vi "Vision_Processing_L_R5.vi"(0 "Current State":T6(ring)=enum."Short Range", 1 "Image Dst":T5=refnum, 2 "Inpute Image":T5=refnum, 3 "Startup Flag":bool, 5 "Current ROI Descriptor":T11={"Global Rectangle"=[0, 0, 320, 240], "Contours"=[{"ID"=enum."External", "Type"=12, "Coordinates"=[0, 0, 320, 240, 0]}]} {"Contours"."Type" items=["No Selection", "Point", "Line", "Rectangle", "Oval", "Polygon", "Freehand Region", "Annulus", "Unused2", "Unused3", "Broken Line", "Freehand Line", "Rotated Rectangle"]}, 6 "Avg Score - Last":dbl=802.5034383138021, 7 "error in (no error)":errorcluster, 8 "Current Settings":T9={"Curve Parameters"={"Extraction Mode"=1, "Edge Threshold"=150, "Edge Filter Size"=0, "Min Length"=25, "Row Search Step Size"=15, "Col Search Step Size"=15, "Max Endpoint Gap"=2, "Closed"=TRUE, "Subpixel"=TRUE}, "Match Mode"={"Rotation"=TRUE, "Scale"=TRUE, "Occlusion"=TRUE, "Reserved"=FALSE, "Reserved"=FALSE, "Reserved"=FALSE}, "Range Settings"=[{"Match Constraints"=0, "Min"=-5.0, "Max"=5.0}, {"Match Constraints"=1, "Min"=20.0, "Max"=150.0}, {"Match Constraints"=2, "Min"=0.0, "Max"=25.0}], "Number of Matches"=1, "Minimum Match Score"=800.0, "SubPixel Accuracy"=TRUE, "Adv. Geometric Match Options 2"=[{"Setup Data Item"=20, "Item Value"=0.0}, {"Setup Data Item"=22, "Item Value"=1.0}]} {"Curve Parameters"."Extraction Mode" items=["Normal", "Uniform Regions"]; "Curve Parameters"."Edge Filter Size" items=["Fine", "Normal", "Contour Tracing"]; "Curve Parameters"."Max Endpoint Gap" min=0; "Curve Parameters"."Col Search Step Size" min=1 max=255 step=1; "Curve Parameters"."Row Search Step Size" min=1 max=255 step=1; "Curve Parameters"."Min Length" min=0; "Curve Parameters"."Edge Threshold" min=1 max=350 step=1; "Range Settings"."Max" format="%.2f"; "Range Settings"."Min" format="%.2f"; "Range Settings"."Match Constraints" items=["Rotation Angle (degrees)", "Scale Factor (%)", "Occlusion (%)"]; "Adv. Geometric Match Options 2"."Setup Data Item" items=["Curve Extraction Mode", "Curve Edge Threshold", "Curve Edge Filter Size", "Min Curve Length", "Curve Row Search Step Size", "Curve Col Search Step Size", "Curve Max Endpoint Gap", "Extract Closed Curves", "Enable Subpixel Curve Extraction", "Enable Correlation Score", "Enable Subpixel Accuracy", "Subpixel Iterations", "Subpixel Tolerance", "Initial Match List Length", "Enable Target Template Curve Score", "Min Match Separation Distance", "Min Match Separation Angle", "Min Match Separation Scale", "Max Match Overlap", "Enable Coarse Result", "Enable Calibration Support", "Enable Contrast Reversal", "Search Strategy", "Refinement Match Factor", "Subpixel Match Factor"]}, 9 "Sub Beacon Search Enable":bool[](array[boolean])=[FALSE, FALSE, FALSE, FALSE, FALSE], 10 "History Data - IN":T4={"Valid Beacon History - in"=[FALSE, FALSE, FALSE, FALSE, FALSE, FALSE, FALSE, FALSE, FALSE, FALSE, FALSE, FALSE, FALSE, FALSE, FALSE, FALSE, FALSE, FALSE, FALSE, FALSE], "Valid Score History"=[916.1194458007812, 0.0, 921.171142578125, 952.2998657226562, 947.6416015625, 946.7607421875, 946.6710815429688, 913.2891235351562, 946.3783569335938, 946.1008911132812, 949.7362060546875, 948.7965087890625, 947.1905517578125, 948.5363159179688, 949.03466796875, 951.10986328125, 800.9814453125, 952.3334350585938, 926.0540161132812, 946.85888671875], "Valid Scale History"=[77.35153198242188, 0.0, 77.18988037109375, 76.20046997070312, 76.42532348632812, 76.47498321533203, 76.45317840576172, 77.11006927490234, 76.4490966796875, 76.39661407470703, 76.34481048583984, 76.36200714111328, 76.56851196289062, 76.3750228881836, 76.43797302246094, 76.20098876953125, 68.23258972167969, 76.18832397460938, 77.75858306884766, 76.44164276123047]} {"Valid Scale History" format="%#_13g"; "Valid Score History" format="%#_13g"}, 13 "Avg Scale - Last":dbl=73.9835688273112, 16 "History Size":i32=20) -> (11 "Avg Scale":dbl=73.9835688273112, 12 "Avg Score":dbl=802.5034383138021, 14 "Tracking Info":T1, 15 "Next Main ROI Descriptor":T2 {"Contours"."Type" items=["No Selection", "Point", "Line", "Rectangle", "Oval", "Polygon", "Freehand Region", "Annulus", "Unused2", "Unused3", "Broken Line", "Freehand Line", "Rotated Rectangle"]}, 17 "Beacon - Scales":sgl[](array[numeric])=[0.0, 0.0, 133.74268, 128.61499, 0.0], 18 "History Data - Out":T3={"Valid Beacon History\nOut"=[FALSE, FALSE, FALSE, FALSE, FALSE, FALSE, FALSE, FALSE, FALSE, FALSE, FALSE, FALSE, FALSE, FALSE, FALSE, FALSE, FALSE, FALSE, FALSE, FALSE], "Valid Score History\nOut"=[916.1194458007812, 0.0, 921.171142578125, 952.2998657226562, 947.6416015625, 946.7607421875, 946.6710815429688, 913.2891235351562, 946.3783569335938, 946.1008911132812, 949.7362060546875, 948.7965087890625, 947.1905517578125, 948.5363159179688, 949.03466796875, 951.10986328125, 800.9814453125, 952.3334350585938, 926.0540161132812, 946.85888671875], "Valid Scale History\nOut"=[77.35153198242188, 0.0, 77.18988037109375, 76.20046997070312, 76.42532348632812, 76.47498321533203, 76.45317840576172, 77.11006927490234, 76.4490966796875, 76.39661407470703, 76.34481048583984, 76.36200714111328, 76.56851196289062, 76.3750228881836, 76.43797302246094, 76.20098876953125, 68.23258972167969, 76.18832397460938, 77.75858306884766, 76.44164276123047]} {"Valid Scale History\nOut" format="%#_13g"; "Valid Score History\nOut" format="%#_13g"}, 19 "Y Coordinates":sgl[](array[numeric])=[0.0, 0.0, 133.74268, 128.61499, 0.0], 20 "Beacons Found":bool[](array[boolean])=[FALSE, FALSE, TRUE, TRUE, FALSE], 21 "X Coordinates":sgl[](array[numeric])=[0.0, 0.0, 162.26208, 213.98871, 0.0], 23 "Lock Status":bool, 24 "Startup Flag - out":bool, 25 "New Settings":T9={"Curve Parameters"={"Extraction Mode"=1, "Edge Threshold"=150, "Edge Filter Size"=0, "Min Length"=25, "Row Search Step Size"=15, "Col Search Step Size"=15, "Max Endpoint Gap"=2, "Closed"=TRUE, "Subpixel"=TRUE}, "Match Mode"={"Rotation"=TRUE, "Scale"=TRUE, "Occlusion"=TRUE, "Reserved"=FALSE, "Reserved"=FALSE, "Reserved"=FALSE}, "Range Settings"=[{"Match Constraints"=0, "Min"=-5.0, "Max"=5.0}, {"Match Constraints"=1, "Min"=20.0, "Max"=150.0}, {"Match Constraints"=2, "Min"=0.0, "Max"=25.0}], "Number of Matches"=1, "Minimum Match Score"=800.0, "SubPixel Accuracy"=TRUE, "Adv. Geometric Match Options 2"=[{"Setup Data Item"=20, "Item Value"=0.0}, {"Setup Data Item"=22, "Item Value"=1.0}]} {"Curve Parameters"."Extraction Mode" items=["Normal", "Uniform Regions"]; "Curve Parameters"."Edge Filter Size" items=["Fine", "Normal", "Contour Tracing"]; "Curve Parameters"."Max Endpoint Gap" min=0; "Curve Parameters"."Col Search Step Size" min=1 max=255 step=1; "Curve Parameters"."Row Search Step Size" min=1 max=255 step=1; "Curve Parameters"."Min Length" min=0; "Curve Parameters"."Edge Threshold" min=1 max=350 step=1; "Range Settings"."Max" format="%.2f"; "Range Settings"."Min" format="%.2f"; "Range Settings"."Match Constraints" items=["Rotation Angle (degrees)", "Scale Factor (%)", "Occlusion (%)"]}, 26 "Next State":T6(ring)=enum."Short Range", 27 "Right Image 2":T5(plugin-control))   [LabVIEW 2015]
uses:
  <vilib>/vision/Image Controls.llb/IMAQ Image.ctl
  <vilib>/vision/Pattern Matching.llb/IMAQ Curve Parameters.ctl
  <vilib>/vision/Pattern Matching.llb/IMAQ Match Range Setting.ctl
panel:
  in  "SR / SCR\nTransition Scale":sgl=100.0
  in  "Score\nCushion- tight":dbl=75.0
  in  "Main ROI Decay\nper Fail (Vertical)":i32=5
  in  "ROI_factor(Horiztonal) SCR":sgl=1.7
  in  "ROI_factor(vertical) SCR":sgl=1.5
  in  "Dumping Range Beacon Filepath**":path=path "/home/lvuser/natinst/bin/BeaconTemplates/SCR_LEFT.png"
  in  "Scale Decay \nFactor":dbl=0.5
  in  "Scale Decay \nFactor":dbl=5.0
  in  "Valid Treshold\nfor Lock":i16=3
  in  "Horiztonall Beacon \nCushion (pixels)":sgl=25.0
  out "New Min Score":dbl=800.0
  out "New Low Scale":dbl=20.0
  out "New high Scale":dbl=150.0
  in  "Absolute\nMinimum Score":dbl=700.0
  in  "Absolute\nMaximum Scale":dbl=300.0
  in  "Absolute\nMinimum Scale":dbl=10.0
  in  "Default No Lock\nSetting Values":T10={"Min Scale"=20.0, "Max Scale"=170.0, "Min Score"=800.0}
  in  "Score\nCushion":dbl=125.0
  in  "Scale \nCushion":dbl=7.0
  in  "LR to SR\nTransition Scale":sgl=80.0
  in  "SR /  LR\nTransition Scale":sgl=80.0
  in  "Timeout \nThrehsold":i32=1000
  in  "Main ROI Decay\nper Fail (Horiztonal)":i32=25
  in  "ROI_factor(Horiztonal) LR":sgl=5.0
  in  "ROI_factor(vertical) LR":sgl=1.5
  in  "ROI_factor(vertical) SR":sgl=2.7
  in  "ROI_factor(Horiztonal) SR":sgl=2.0
  out "Current  Score":sgl=916.11945
  out "Current  Scale":sgl=77.35153
  in  "Fail Count - In":i32
  in  "Sub Beacon Template File Path - ARRAY":path[](array[path])=[path "/home/lvuser/natinst/bin/BeaconTemplates/Sub1.png", path "/home/lvuser/natinst/bin/BeaconTemplates/Sub2.png", path "/home/lvuser/natinst/bin/BeaconTemplates/Sub3.png", path "/home/lvuser/natinst/bin/BeaconTemplates/Sub4.png", path "/home/lvuser/natinst/bin/BeaconTemplates/Sub5.png"]
  in  "Short Range Template FIle Path":path=path "/home/lvuser/natinst/bin/BeaconTemplates/SR_Left.png"
  in  "Long Range Main\nBeacon File Path":path=path "/home/lvuser/natinst/bin/BeaconTemplates/LR_Main.png"
  # "INPUTS"
  # "FILE PATHS"
  # "CONFIG"
  # "OUTPUTS"
  # "************"
  # "Range"
  # "Range"
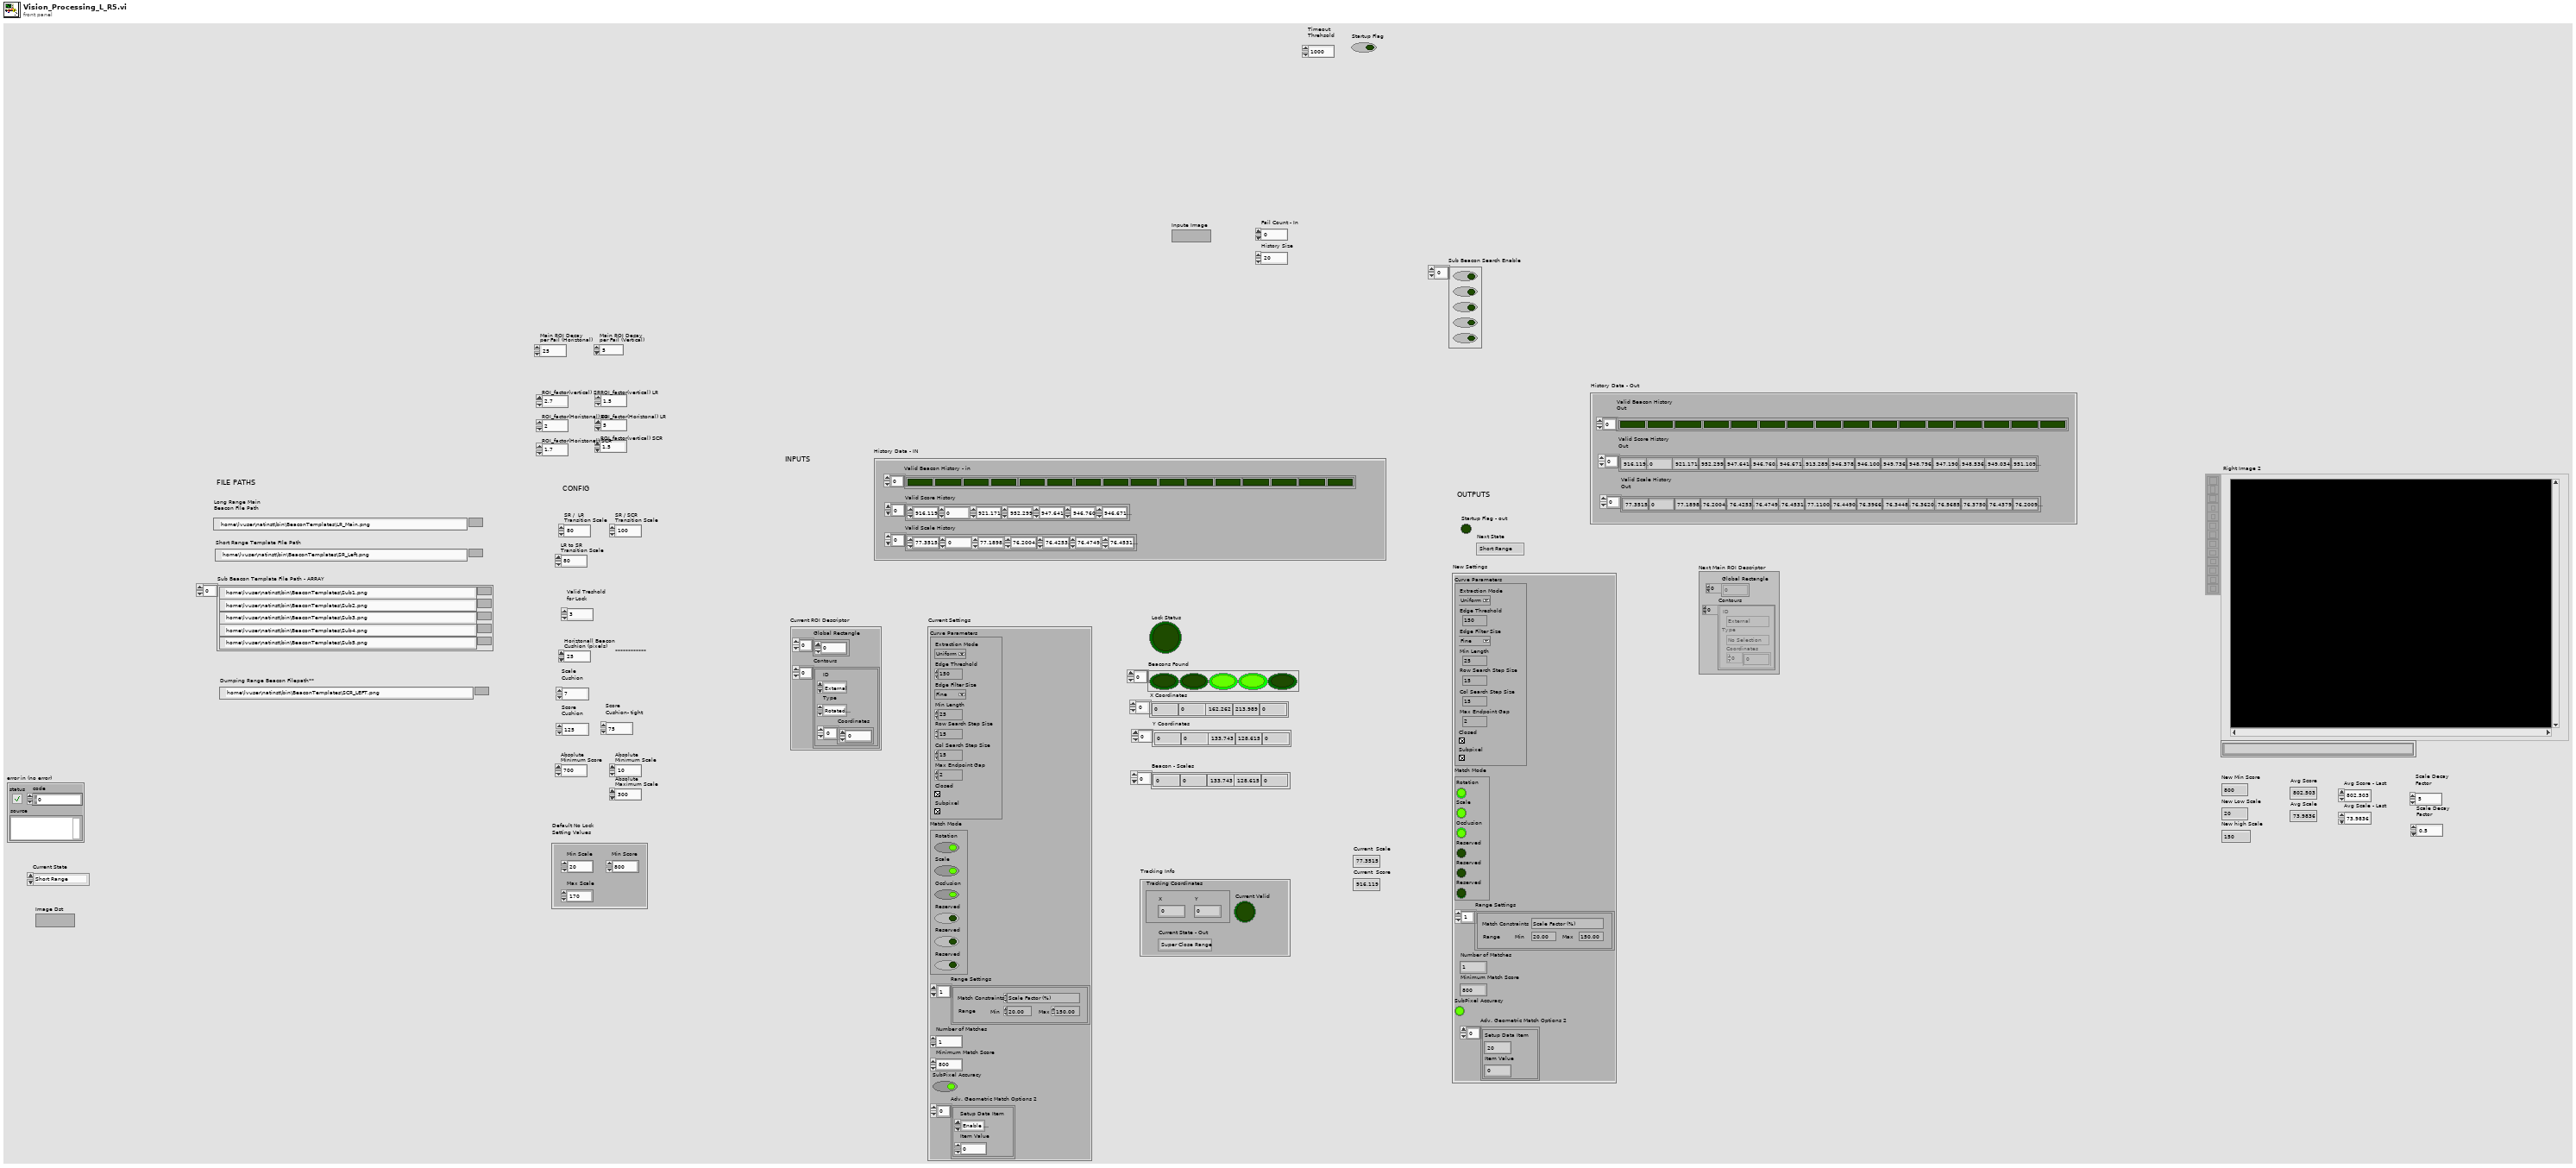
[diagram p1: front panel]
types:
  T1 = cluster{"Tracking Coordinates":cluster{"X":dbl, "Y":dbl}, "Current Valid":bool, "Current State - Out":enum16{"Super Close Range", "Short Range", "Long Range"}}
  T2 = typedef "ROI Descriptor" = cluster{"Global Rectangle":i32[], "Contours":cluster{"ID":enum32{"External", "Internal"}, "Type":u32, "Coordinates":i32[]}[]}
  T3 = cluster{"Valid Beacon History\nOut":bool[], "Valid Score History\nOut":dbl[], "Valid Scale History\nOut":dbl[]}
  T4 = cluster{"Valid Beacon History - in":bool[], "Valid Score History":dbl[], "Valid Scale History":dbl[]}
  T5 = typedef "IMAQ Image.ctl" = refnum<image>
  T6 = enum16{"Super Close Range", "Short Range", "Long Range"}
  T7 = typedef "IMAQ Curve Parameters.ctl" = cluster{"Extraction Mode":u32, "Edge Threshold":i32, "Edge Filter Size":u32, "Min Length":i32, "Row Search Step Size":i32, "Col Search Step Size":i32, "Max Endpoint Gap":i32, "Closed":bool, "Subpixel":bool}
  T8 = typedef "IMAQ Match Range Setting.ctl" = cluster{"Match Constraints":u32, "Min":dbl, "Max":dbl}
  T9 = cluster{"Curve Parameters":T7, "Match Mode":cluster{"Rotation":bool, "Scale":bool, "Occlusion":bool, "Reserved":bool, "Reserved":bool, "Reserved":bool}, "Range Settings":T8[], "Number of Matches":i32, "Minimum Match Score":sgl, "SubPixel Accuracy":bool, "Adv. Geometric Match Options 2":cluster{"Setup Data Item":u16, "Item Value":dbl}[]}
  T10 = cluster{"Min Scale":dbl, "Max Scale":dbl, "Min Score":dbl}
  T11 = cluster{"Global Rectangle":i32[], "Contours":cluster{"ID":enum32{"External", "Internal"}, "Type":u32, "Coordinates":i32[]}[]}
  T12 = typedef "IMAQ GM Match Report.ctl" = cluster{"Position":cluster{"x":sgl, "y":sgl}, "Angle":sgl, "Scale":sgl, "Score":sgl, "Bounding Box":cluster{"x":sgl, "y":sgl}[], "Contrast Reversed":bool, "Occlusion %":sgl, "Template Target Curve Score":sgl, "Target Template Curve Score":sgl, "Correlation Score":sgl}
  T13 = cluster{"Matches (Geometric Matching 1)[0]":T12, "Matches (Geometric Matching 1)[1]":T12, "Matches (Geometric Matching 1)[2]":T12, "Matches (Geometric Matching 1)[3]":T12, "Matches (Geometric Matching 1)[4]":T12, "Matches (Geometric Matching 1)[5]":T12, "Matches (Geometric Matching 1)[6]":T12, "Matches (Geometric Matching 1)[7]":T12, "Matches (Geometric Matching 1)[8]":T12}
  T14 = cluster{"Bounding Box[0]":cluster{"x":sgl, "y":sgl}, "Bounding Box[1]":cluster{"x":sgl, "y":sgl}, "Bounding Box[2]":cluster{"x":sgl, "y":sgl}, "Bounding Box[3]":cluster{"x":sgl, "y":sgl}, "Bounding Box[4]":cluster{"x":sgl, "y":sgl}, "Bounding Box[5]":cluster{"x":sgl, "y":sgl}, "Bounding Box[6]":cluster{"x":sgl, "y":sgl}, "Bounding Box[7]":cluster{"x":sgl, "y":sgl}, "Bounding Box[8]":cluster{"x":sgl, "y":sgl}}
  T15 = cluster{"Position":cluster{"x":sgl, "y":sgl}, bool, "Current State":enum16{"Super Close Range", "Short Range", "Long Range"}}
  T16 = typedef "IMAQ Rectangle" = cluster{"Left":i32, "Top":i32, "Right":i32, "Bottom":i32, "Rotation":dbl}
  T17 = cluster{"index":u32, "Min Scale":dbl, "Max Scale":dbl}
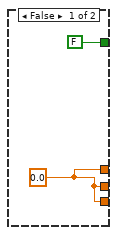
[diagram p2: hidden frame]
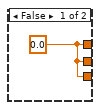
[diagram p3: hidden frame]
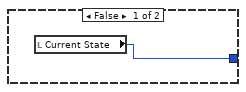
[diagram p7: hidden frame]
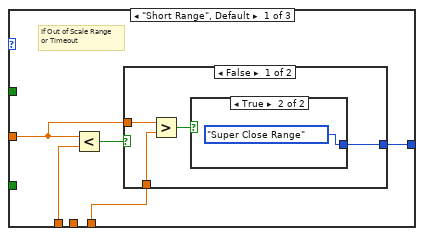
[diagram p8: hidden frame]
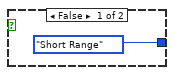
[diagram p9: hidden frame]
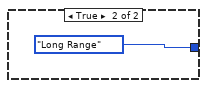
[diagram p10: hidden frame]
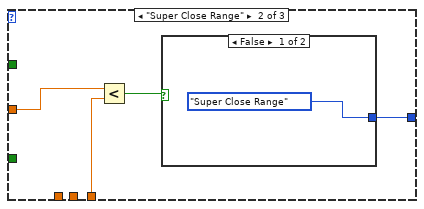
[diagram p11: hidden frame]
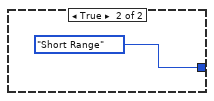
[diagram p12: hidden frame]
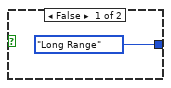
[diagram p13: hidden frame]
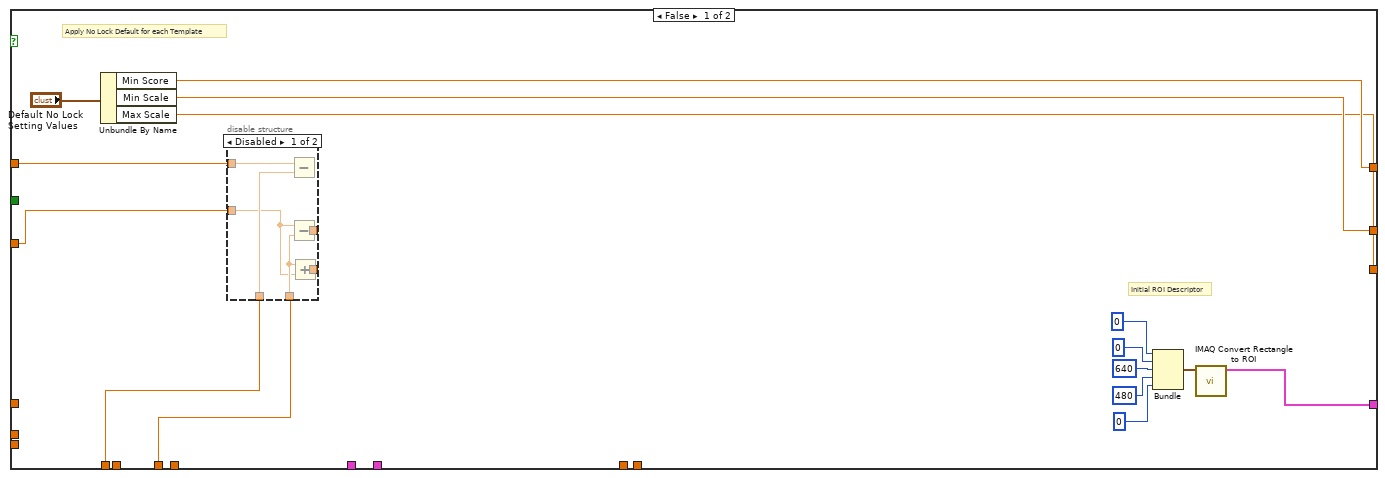
[diagram p15: hidden frame]
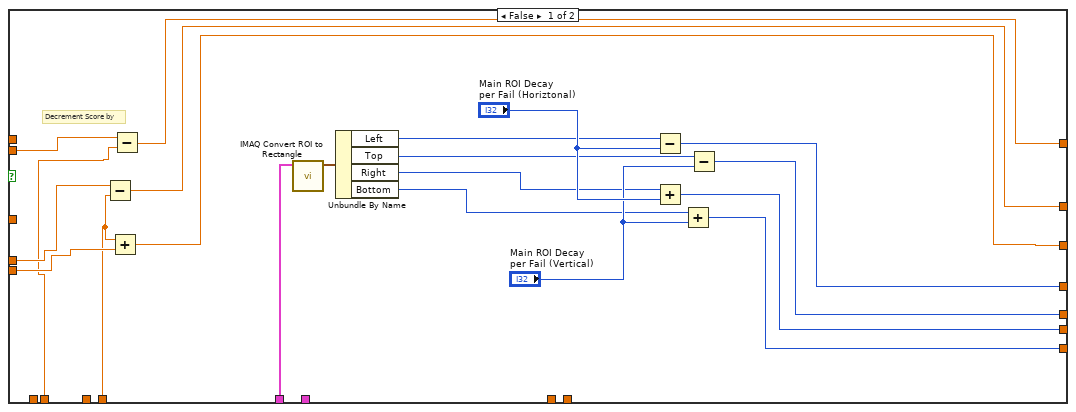
[diagram p17: hidden frame]
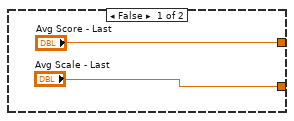
[diagram p18: hidden frame]
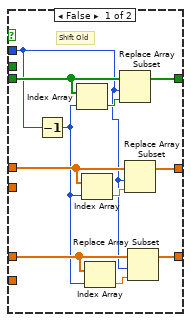
[diagram p20: hidden frame]
diagram:
  (unwired) enum16{"Short Range", "Long Range"}."Short Range"
  # "Next Settings"
  n1 = flat-sequence {
    tunnel: [w8] -> w3
    tunnel: [w7] -> w2
    tunnel: ["Image Dst"] -> w1
    tunnel: w3 -> [w131]
    tunnel: w2 -> [w129]
    tunnel: w1 -> [w130]
    frame #0 {
      # "APPLY FILTERING"
      n2 = call "Camera - Filtering"("Image In"="Inpute Image", "Image Dst"="Image Dst", "error in"="error in (no error)") -> ("Image Out"=w8:T5, "error out"=w7:errorcluster)  [unwired: 23 in]
    }
    frame #1 {
      w90 = u32 1 ("index")
      w111 = u8 5
      # "Current is Valid"
      # "Update Tracking Coordinates"
      # "CURRENT VALID"
      # "*************"
      # "Beacon - Y"
      # "Beacon - X"
      # "Beacons Found"
      # "Build ROI for Individual Beacons Based on Main Bounding Box"
      # "Starting X Lower Bound"
      # "Length of\nIndividual Beacon ROI"
      # "Length of Bounding Box"
      # "Force SCR if Flagged"
      # "Choose ROI Factor based on Next State"
      # "Current Match"
      # "Current ROI"
      # "Image Lock"
      # "Force SR on Startup"
      # "Valid History"
      # "Draw ROI and stuff on outputi mage"
      # "Pull Down Startup IF Already True and Lock\nOtherwise don't update"
      # "Next Settings"
      # "Apply Limits to Settings"
      # "Scale"
      # "Min Score"
      # "Lower Scale"
      # "Upper Scale"
      # "Current Settings"
      # "Current Min\n& Max Scale"
      # "Current Valid"
      # "Update Search Settings"
      # "Update Template State"
      # "Calculate Average Scale/Score"
      # "max avg"
      # "Min Required to use avarage"
      # "Valid  Ccount\n(up to 3)"
      # "****# of previous in history that must be true\nin order for position to be considered \"locked\""
      # "Update Shift Arrays"
      # "# of Beacons Found to be valid"
      # "# of beacons"
      # "Matches"
      # "image out"
      n3 = Select(t=T6."Short Range", s="Startup Flag", f="Current State") -> (s? t:f=w9:T6)
      n4 = case shown="\"Super Close Range\", Default" w9 {
        tunnel: w131 -> [w394 w428 w461]
        tunnel: w130 -> [w393 w427 w460]
        tunnel: "Current ROI Descriptor" -> [w391 w425 w459]
        tunnel: "Current Settings" -> [w390 w424 w458]
        tunnel: [w386 w420 w454] -> w47
        tunnel: [w387 w419 w453] -> w70
        tunnel: [w388 w417 w451] -> w120
        tunnel: w129 -> [w392 _ w450]
        tunnel: "Sub Beacon Search Enable" -> [w395 w418 w449]
        tunnel: [2.0 sgl 3.0 ("y") sgl 5.0 ("y")] -> w127
        tunnel: [w384 w415 w447] -> w126
        tunnel: [1 2 3] -> w121
        frame "Super Close Range", Default {
          # "**Make sure this selects the \nbeacon used for close range!!!"
          n5 = call "Dumping Range"("Image In"=w394, "Image Dst"=w393, "ROI Descriptor (Geometric Matching 1)"=w391, "Settings (Geometric Matching 1)"=w390, "Template File Path (Geometric Matching 1)"="Dumping Range Beacon Filepath**", "error in"=w392) -> ("Image Out"=w387:T5, "Matches (Geometric Matching 1)"=w386:T12[], "Number of Matches (Geometric Matching 1)"=w383:i32, "error out"=w384:errorcluster)  [unwired: 18 in]
          n6 = Equal?(x=w383, y=1) -> (x = y?=w381:bool)
          n7 = case shown="True" w381 {
            tunnel: w395 -> [w404 w407]
            tunnel: [w397 w408] -> w388
            frame False {
              w398 = FALSE
              # "F"
              # "No Main Found,\nDon't Search any Subs"
              n8 = Replace Array Subset(array=w404, new element #1=w398, index #1=0 ("y"), new element #2=w398, index #2=1 ("y"), new element #3=w398, index #3=2 ("y"), new element #4=w398, index #4=3 ("y"), new element #5=w398, index #5=4 ("y")) -> (w397:bool[])
            }
            frame True {
              w406 = TRUE
              w405 = FALSE
              # "Search for MIDDLE Beacons"
              n9 = Replace Array Subset(array=w407, new element #1=w406, index #1=0 ("y"), new element #2=w406, index #2=1 ("y"), new element #3=w405, index #3=2 ("y"), new element #4=w405, index #4=3 ("y"), new element #5=w405, index #5=4 ("y")) -> (w408:bool[])
            }
          }
        }
        frame "Short Range" {
          n10 = call "Short Range"("Image In"=w428, "Image Dst"=w427, "ROI Descriptor (Geometric Matching 1)"=w425, "Settings (Geometric Matching 1)"=w424, "Template File Path (Geometric Matching 1)"="Short Range Template FIle Path") -> ("Image Out"=w419:T5, "Matches (Geometric Matching 1)"=w420:T12[], "Number of Matches (Geometric Matching 1)"=w421:i32, "error out"=w415:errorcluster)  [unwired: 19 in]
          n11 = Equal?(x=w421, y=1) -> (x = y?=w422:bool)
          n12 = case shown="True" w422 {
            tunnel: w418 -> [w436 w439]
            tunnel: [w429 w440] -> w417
            frame False {
              w430 = FALSE
              # "F"
              # "No Main Found,\nDon't Search any Subs"
              n13 = Replace Array Subset(array=w436, new element #1=w430, index #1=0 ("y"), new element #2=w430, index #2=1 ("y"), new element #3=w430, index #3=2 ("y"), new element #4=w430, index #4=3 ("y"), new element #5=w430, index #5=4 ("y")) -> (w429:bool[])
            }
            frame True {
              w438 = TRUE
              w437 = FALSE
              # "Search for specific Beacons"
              n14 = Replace Array Subset(array=w439, new element #1=w438, index #1=0 ("y"), new element #2=w438, index #2=1 ("y"), new element #3=w438, index #3=2 ("y"), new element #4=w437, index #4=3 ("y"), new element #5=w437, index #5=4 ("y")) -> (w440:bool[])
            }
          }
        }
        frame "Long Range" {
          n15 = call "Long Range"("Image In"=w461, "Image Dst"=w460, "ROI Descriptor (Geometric Matching 1)"=w459, "Settings (Geometric Matching 1)"=w458, "Template File Path (Geometric Matching 1)"="Long Range Main\nBeacon File Path", "error in"=w450) -> ("Image Out"=w453:T5, "Matches (Geometric Matching 1)"=w454:T12[], "Number of Matches (Geometric Matching 1)"=w456:i32, "error out"=w447:errorcluster)  [unwired: 18 in]
          n16 = Equal?(x=w456, y=1) -> (x = y?=w452:bool)
          n17 = case shown="True" w452 {
            tunnel: w449 -> [w469 w471]
            tunnel: [w462 w470] -> w451
            frame False {
              w463 = FALSE
              # "F"
              # "No Main Found,\nDon't Search any Subs"
              n18 = Replace Array Subset(array=w469, new element #1=w463, index #1=0 ("y"), new element #2=w463, index #2=1 ("y"), new element #3=w463, index #3=2 ("y"), new element #4=w463, index #4=3 ("y"), new element #5=w463, index #5=4 ("y")) -> (w462:bool[])
            }
            frame True {
              w472 = TRUE
              # "T"
              # "Search for ALL Beacons"
              n19 = Replace Array Subset(array=w471, new element #1=w472, index #1=0 ("y"), new element #2=w472, index #2=1 ("y"), new element #3=w472, index #3=2 ("y"), new element #4=w472, index #4=3 ("y"), new element #5=w472, index #5=4 ("y")) -> (w470:bool[])
            }
          }
        }
      }
      n20 = Array To Cluster(array=w47) -> (cluster=w37:T13)
      n21 = Unbundle By Name(w37) -> ("Matches (Geometric Matching 1)[0].Position"=w11:cluster{"x":sgl, "y":sgl}, "Matches (Geometric Matching 1)[0].Bounding Box"=w35:cluster{"x":sgl, "y":sgl}[], "Matches (Geometric Matching 1)[0].Scale"=w69:sgl, "Matches (Geometric Matching 1)[0].Score"=w81:sgl)
      "Current  Scale" <- w69
      "Current  Score" <- w81
      n22 = Array To Cluster(array=w35) -> (cluster=w36:T14)
      n23 = Unbundle By Name(w36) -> ("Bounding Box[0].x"=w26:sgl, "Bounding Box[0].y"=w25:sgl, "Bounding Box[2].x"=w24:sgl, "Bounding Box[2].y"=w23:sgl)
      n24 = Bundle("x"=w26, "y"=w25, "x"=w24, "y"=w23) -> (w21:cluster{"x":sgl, "y":sgl, "x":sgl, "y":sgl})  [unwired: 1 in]
      n25 = call "IMAQ Overlay Rectangle"("Rectangle"=w21, "Image"=w70) -> ("Image Out"=w22:T5)  [unwired: 8 in, 1 out]
      n26 = Subtract(x=w24, y=w26) -> (x-y=w30:sgl)
      n27 = Divide(x=w30, y=w127) -> (x/y=w32:dbl)
      n28 = Multiply(x="Horiztonall Beacon \nCushion (pixels)", y=w69) -> (x*y=w20:sgl)
      n29 = Divide(x=w20, y=sgl 100.0) -> (x/y=w17:sgl)
      n30 = Subtract(x=w25, y=w17) -> (x-y=w33:sgl)
      n31 = Add(x=w17, y=w23) -> (x+y=w34:sgl)
      n32 = for {
        N: 5 -> [_]
        tunnel: w120 -> [w174] mode=indexing
        shift-right: [w168] -> _
        shift-left: w26 -> [w173]
        tunnel: w32 -> [w172]
        tunnel: w33 -> [w165]
        tunnel: w34 -> [w164]
        tunnel: [w171] -> w28 mode=indexing
        tunnel: w17 -> [w166]
        # "Divide Bounding Box"
        # "Upper Bound of Current is\nLower Bound for Next"
        n33 = case shown="True" w174 {
          tunnel: w173 -> [w175 w176]
          tunnel: w172 -> [_ w178]
          tunnel: [w175 w177] -> w168
          tunnel: [w175 w176] -> w170
          frame False {
            # "Don't Care"
          }
          frame True {
            # "X Lower Bound"
            n34 = Add(x=w176, y=w178) -> (x+y=w177:dbl)
          }
        }
        n35 = Subtract(x=w170, y=w166) -> (x-y=w169:dbl)
        n36 = Add(x=w168, y=w166) -> (x+y=w167:dbl)
        n37 = call "Bound_RO_R_R0I.vi"("Bottom Right - Y"=w164, "Right - X"=w167, "Top Left - Y"=w165, "Top  Left - x"=w169) -> ("ROI Descriptor"=w171:T2)  [unwired: 7 in]
      }
      n38 = for {
        N: 5 -> [_]
        tunnel: w70 -> [w143]
        tunnel: w126 -> [w142]
        tunnel: w28 -> [w135] mode=indexing
        tunnel: "Sub Beacon Template File Path - ARRAY" -> [w141] mode=indexing
        tunnel: [w140] -> w125 mode=indexing
        tunnel: [w139] -> w124 mode=indexing
        tunnel: [w138] -> w112 mode=indexing
        tunnel: w120 -> [w137] mode=indexing
        tunnel: "Current Settings" -> [w136]
        shift-right: [w133] -> w71
        shift-left: w22 -> [w134]
        tunnel: [w132] -> w60 mode=indexing
        n39 = case shown="True" w137 {
          tunnel: w143 -> [_ w157]
          tunnel: w142 -> [_ w156]
          tunnel: w135 -> [_ w155]
          tunnel: w141 -> [_ w154]
          tunnel: [w144 w150] -> w140
          tunnel: [w144 w149] -> w139
          tunnel: [FALSE w148] -> w138
          tunnel: w136 -> [_ w147]
          tunnel: [w144 w146] -> w132
          frame False {
            w144 = sgl 0.0 ("x")
          }
          frame True {
            n40 = call "Sub Beacon Pattern Match"("Image In"=w157, "ROI Descriptor (Geometric Matching 1)"=w155, "Settings (Geometric Matching 1)"=w147, "Template File Path (Geometric Matching 1)"=w154, "error in"=w156) -> ("Matches (Geometric Matching 1)"=w151:T12[], "Number of Matches (Geometric Matching 1)"=w152:i32)  [unwired: 19 in, 2 out]
            n41 = Equal?(x=w152, y=1) -> (x = y?=w148:bool)
            n42 = case shown="True" w148 {
              tunnel: w151 -> [_ w162]
              tunnel: [w158 w161] -> w150
              tunnel: [w158 w160] -> w149
              tunnel: [w158 w159] -> w146
              frame False {
                w158 = sgl 0.0 ("x")
              }
              frame True {
                n43 = Array To Cluster(array=w162) -> (cluster=w163:T13)
                n44 = Unbundle By Name(w163) -> ("Matches (Geometric Matching 1)[0].Position.x"=w161:sgl, "Matches (Geometric Matching 1)[0].Position.y"=w160:sgl, "Matches (Geometric Matching 1)[0].Scale"=w159:sgl)
              }
            }
          }
        }
        n45 = call "IMAQ Overlay ROI"("ROI Descriptor"=w135, "Image"=w134) -> ("Image Out"=w133:T5)  [unwired: 8 in, 1 out]
      }
      "Beacons Found" <- w112
      "X Coordinates" <- w125
      "Y Coordinates" <- w124
      "Beacon - Scales" <- w60
      n46 = Boolean To (0,1)(Boolean=w112) -> (0, 1=w122:i16[])
      n47 = Add Array Elements(numeric array=w122) -> (sum=w123:i16)
      n48 = Greater Or Equal?(x=w123, y=w121) -> (x >= y?=w10:bool)
      n49 = case shown="False" w10 {
        tunnel: "Fail Count - In" -> [w379 _]
        tunnel: [w378 u16 0] -> w104
        frame False {
          n50 = Increment(x=w379) -> (x+1=w378:i32)
        }
        frame True {
          # "reset fail count"
        }
      }
      n51 = Unbundle By Name("History Data - IN") -> ("Valid Beacon History - in"=w67:bool[], "Valid Score History"=w66:dbl[], "Valid Scale History"=w65:dbl[])
      n52 = Greater?(x=w104, y="Timeout \nThrehsold") -> (0:w13:bool)
      n53 = Decrement(x="History Size") -> (x-1=w118:i32)
      n54 = for {
        N: "History Size" -> [_]
        shift-right: [w356] -> w64
        shift-left: w67 -> [w344]
        tunnel: w118 -> [w352]
        shift-right: [w349] -> w63
        shift-left: w66 -> [w351]
        shift-right: [w348] -> w62
        shift-left: w65 -> [w350]
        tunnel: w81 -> [w347]
        tunnel: w69 -> [w346]
        tunnel: w10 -> [w345]
        i -> [w355]
        # "Reverse Index"
        n55 = Subtract(x=w352, y=w355) -> (x-y=w353:i32)
        n56 = Equal To 0?(x=w353) -> (x = 0?=w354:bool)
        n57 = case shown="True" w354 {
          tunnel: w353 -> [w357 w376]
          tunnel: w344 -> [w367 w369]
          tunnel: [w365 w368] -> w356
          tunnel: w345 -> [_ w377]
          tunnel: w351 -> [w362 w375]
          tunnel: w350 -> [w361 w374]
          tunnel: [w360 w372] -> w349
          tunnel: [w359 w373] -> w348
          tunnel: w347 -> [_ w371]
          tunnel: w346 -> [_ w370]
          frame False {
            # "Shift Old"
            n58 = Decrement(x=w357) -> (x-1=w358:i32)
            n59 = Index Array(array=w367, index=w358) -> (element=w366:bool)
            n60 = Index Array(array=w362, index=w358) -> (element=w364:dbl)
            n61 = Index Array(array=w361, index=w358) -> (element=w363:dbl)
            n62 = Replace Array Subset(array=w367, new element=w366, index=w357) -> (w365:bool[])
            n63 = Replace Array Subset(array=w362, new element=w364, index=w357) -> (w360:dbl[])
            n64 = Replace Array Subset(array=w361, new element=w363, index=w357) -> (w359:dbl[])
          }
          frame True {
            # "Scale"
            # "Score"
            # "Valid"
            # "insert New"
            n65 = Replace Array Subset(array=w375, new element=w371, index=w376) -> (w372:dbl[])
            n66 = Replace Array Subset(array=w374, new element=w370, index=w376) -> (w373:dbl[])
            n67 = Replace Array Subset(array=w369, new element=w377, index=w376) -> (w368:bool[])
          }
        }
      }
      n68 = Boolean To (0,1)(Boolean=w64) -> (0, 1=w116:i16[])
      n69 = Bundle("Valid Beacon History - in"=w64, "Valid Score History"=w63, "Valid Scale History"=w62) -> (→"History Data - Out":T4)  [unwired: 1 in]
      n70 = Add Array Elements(numeric array=w116) -> (sum=w117:i16)
      n71 = Greater Or Equal?(x=w117, y="Valid Treshold\nfor Lock") -> (x >= y?=w82:bool)
      "Lock Status" <- w82
      n72 = Initialize Array(u8 0, w111) -> (w114:u8[])
      n73 = while {
        shift-right: [w327] -> w109
        shift-left: w114 -> [w329]
        tunnel: w64 -> [w335] mode=indexing
        shift-right: [w333] -> w107
        shift-left: u8 0 -> [w336]
        tunnel: "History Size" -> [w334]
        tunnel: w111 -> [w326]
        i -> [w328]
        stop <- w330 stop-if-true
        # "Grab Last 2 Valid Indexes"
        n74 = case shown="True" w335 {
          tunnel: w336 -> [w338 w340]
          tunnel: [w338 w343] -> w333
          tunnel: w329 -> [w337 w342]
          tunnel: w328 -> [_ w341]
          tunnel: [w337 w339] -> w327
          frame False {
          }
          frame True {
            # "Update Index\nto use"
            # "Increment\nValid Count"
            n75 = Replace Array Subset(array=w342, new element=w341, index=w340) -> (w339:u8[])
            n76 = Increment(x=w340) -> (x+1=w343:u8)
          }
        }
        n77 = Greater?(x=w328, y=w334) -> (0:w331:bool)
        n78 = Greater Or Equal?(x=w333, y=w326) -> (x >= y?=w332:bool)
        n79 = Or(x=w332, y=w331) -> (x .or. y?=w330:bool)
      }
      n80 = Greater?(x=w107, y=u8 2) -> (0:w108:bool)
      n81 = case shown="True" w108 {
        tunnel: w107 -> [_ w310]
        tunnel: w109 -> [_ w316]
        tunnel: w63 -> [_ w315]
        tunnel: w62 -> [_ w314]
        tunnel: ["Avg Score - Last" w308] -> w78
        tunnel: ["Avg Scale - Last" w307] -> w79
        frame False {
        }
        frame True {
          w313 = 0.0
          n82 = for {
            N: w310 -> [_]
            tunnel: w316 -> [w323] mode=indexing
            tunnel: w315 -> [w325]
            tunnel: w314 -> [w324]
            shift-right: [w321] -> w312
            shift-left: w313 -> [w319]
            shift-right: [w322] -> w311
            shift-left: w313 -> [w318]
            # "Fetch Last Valid Values"
            n83 = Index Array(array=w325, index=w323) -> (element=w320:dbl)
            n84 = Index Array(array=w324, index=w323) -> (element=w317:dbl)
            n85 = Add(x=w320, y=w319) -> (x+y=w321:dbl)
            n86 = Add(x=w317, y=w318) -> (x+y=w322:dbl)
          }
          n87 = To Double Precision Float(number=w310) -> (double precision float=w309:dbl)
          n88 = Divide(x=w312, y=w309) -> (x/y=w308:dbl)
          n89 = Divide(x=w311, y=w309) -> (x/y=w307:dbl)
        }
      }
      "Avg Score" <- w78
      "Avg Scale" <- w79
      n90 = Bundle("Position"=w11, w10, "Current State"=w9) -> (→"Tracking Info":T15)  [unwired: 1 in]
      n91 = case shown="True" w82 {
        tunnel: w13 -> [_ w192]
        tunnel: "SR /  LR\nTransition Scale" -> [_ w191]
        tunnel: "LR to SR\nTransition Scale" -> [_ w190]
        tunnel: w79 -> [_ w189]
        tunnel: w82 -> [_ w188]
        tunnel: [w185 w187] -> w14
        tunnel: "SR / SCR\nTransition Scale" -> [_ w186]
        frame False {
          n92 = local read "Current State"() -> (w185:T6)
        }
        frame True {
          # "Timeout"
          # "Image Lock"
          n93 = local read "Current State"() -> (w193:T6)
          n94 = case shown="\"Long Range\"" w193 {
            tunnel: w188 -> [_ _ _]
            tunnel: w189 -> [w195 w208 w214]
            tunnel: w192 -> [_ _ _]
            tunnel: w191 -> [w198 _ _]
            tunnel: w190 -> [_ _ w213]
            tunnel: [w196 w206 w212] -> w187
            tunnel: w186 -> [w194 w209 _]
            frame "Short Range", Default {
              # "If Out of Scale Range\nor Timeout"
              n95 = Less?(x=w195, y=w198) -> (x < y?=w197:bool)
              n96 = case shown="False" w197 {
                tunnel: [w202 T6."Long Range"] -> w196
                tunnel: w195 -> [w200 _]
                tunnel: w194 -> [w199 _]
                frame False {
                  n97 = Greater?(x=w200, y=w199) -> (0:w201:bool)
                  n98 = case shown="True" w201 {
                    tunnel: [T6."Short Range" T6."Super Close Range"] -> w202
                    frame False {
                    }
                    frame True {
                    }
                  }
                }
                frame True {
                }
              }
            }
            frame "Super Close Range" {
              n99 = Less?(x=w208, y=w209) -> (x < y?=w207:bool)
              n100 = case shown="False" w207 {
                tunnel: [T6."Super Close Range" T6."Short Range"] -> w206
                frame False {
                }
                frame True {
                }
              }
            }
            frame "Long Range" {
              # "If Out of Scale Range\nor Timeout"
              n101 = Greater?(x=w214, y=w213) -> (0:w215:bool)
              n102 = case shown="True" w215 {
                tunnel: [T6."Long Range" T6."Short Range"] -> w212
                frame False {
                }
                frame True {
                }
              }
            }
          }
        }
      }
      "Next State" <- w14
      n103 = Unbundle By Name("Current Settings") -> ("Minimum Match Score"=w101:sgl, "Range Settings"=w87:T8[])
      n104 = case shown="\"Short Range\"" w14 {
        tunnel: "ROI_factor(vertical) SR" -> [_ _ w184]
        tunnel: "ROI_factor(Horiztonal) SR" -> [_ _ w183]
        tunnel: "ROI_factor(vertical) LR" -> [_ w182 _]
        tunnel: "ROI_factor(Horiztonal) LR" -> [_ w181 _]
        tunnel: "ROI_factor(vertical) SCR" -> [w180 _ _]
        tunnel: "ROI_factor(Horiztonal) SCR" -> [w179 _ _]
        tunnel: [w180 w182 w184] -> w40
        tunnel: [w179 w181 w183] -> w39
        frame "Super Close Range", Default {
        }
        frame "Long Range" {
        }
        frame "Short Range" {
        }
      }
      n105 = Index Array(array=w87, index=u32 1) -> (element=w100:T8)
      n106 = Unbundle(w100) -> ("Min"=w98:dbl, "Max"=w97:dbl)  [unwired: 1 out]
      n107 = case shown="True" w82 {
        tunnel: w10 -> [_ w262]
        tunnel: w78 -> [w231 w261]
        tunnel: w79 -> [w230 w260]
        tunnel: w101 -> [_ w259]
        tunnel: w98 -> [_ w258]
        tunnel: w97 -> [_ w257]
        tunnel: [w229 w248] -> w88
        tunnel: [w228 w247] -> w51
        tunnel: [w227 w246] -> w52
        tunnel: "Scale \nCushion" -> [w233 w256]
        tunnel: "Score\nCushion" -> [w232 w255]
        tunnel: "Scale Decay \nFactor" -> [_ w254]
        tunnel: "Scale Decay \nFactor" -> [_ w253]
        tunnel: "Current ROI Descriptor" -> [_ w249]
        tunnel: w47 -> [_ w250]
        tunnel: w40 -> [_ w252]
        tunnel: w39 -> [_ w251]
        tunnel: [w220 w245] -> w38
        frame False {
          # "Initial ROI Descriptor"
          # "Apply No Lock Default for each Template"
          n108 = Unbundle By Name("Default No Lock\nSetting Values") -> ("Min Score"=w229:dbl, "Min Scale"=w228:dbl, "Max Scale"=w227:dbl)
          n109 = disable-structure shown="Disabled" {
            disable-tunnel: [w240 _] -> _
            disable-tunnel: [w239 _] -> _
            disable-tunnel: w233 -> [w238 _]
            disable-tunnel: w232 -> [w237 _]
            disable-tunnel: w231 -> [w236 _]
            disable-tunnel: w230 -> [w235 _]
            frame Disabled {
              n110 = Subtract(x=w236, y=w237) -> ()  [unwired: 1 out]
              n111 = Subtract(x=w235, y=w238) -> (x-y=w240:dbl)
              n112 = Add(x=w238, y=w235) -> (x+y=w239:dbl)
            }
            frame Enabled {
            }
          }
          n113 = Bundle(0, 0, 640, 480, 0) -> (w226:cluster{i32, i32, i32, i32, i32})  [unwired: 1 in]
          n114 = call "IMAQ Convert Rectangle to ROI"("Rectangle"=w226) -> ("ROI Descriptor"=w220:T2)  [unwired: 8 in, 1 out]
        }
        frame True {
          # "Apply Limits to ROI"
          n115 = case shown="True" w262 {
            tunnel: w261 -> [_ w304]
            tunnel: [w277 w300] -> w248
            tunnel: w260 -> [_ w303]
            tunnel: [w276 w299] -> w247
            tunnel: [w275 w298] -> w246
            tunnel: w258 -> [w282 _]
            tunnel: w257 -> [w281 _]
            tunnel: w259 -> [w280 _]
            tunnel: w256 -> [_ w302]
            tunnel: w255 -> [_ w301]
            tunnel: w254 -> [w279 _]
            tunnel: w253 -> [w278 _]
            tunnel: w252 -> [_ w289]
            tunnel: w251 -> [_ w288]
            tunnel: w250 -> [_ w287]
            tunnel: [w266 w286] -> w244
            tunnel: [w265 w285] -> w243
            tunnel: [w264 w284] -> w242
            tunnel: [w263 w283] -> w241
            tunnel: w249 -> [w273 _]
            frame False {
              # "Decrement Score by"
              n116 = Subtract(x=w282, y=w278) -> (x-y=w276:dbl)
              n117 = Add(x=w278, y=w281) -> (x+y=w275:dbl)
              n118 = Subtract(x=w280, y=w279) -> (x-y=w277:dbl)
              n119 = call "IMAQ Convert ROI to Rectangle"("ROI Descriptor"=w273) -> ("Rectangle"=w274:T16)  [unwired: 8 in, 1 out]
              n120 = Unbundle By Name(w274) -> ("Left"=w270:i32, "Top"=w269:i32, "Right"=w268:i32, "Bottom"=w267:i32)
              n121 = Subtract(x=w270, y="Main ROI Decay\nper Fail (Horiztonal)") -> (x-y=w266:i32)
              n122 = Add(x=w268, y="Main ROI Decay\nper Fail (Horiztonal)") -> (x+y=w264:i32)
              n123 = Add(x=w267, y="Main ROI Decay\nper Fail (Vertical)") -> (x+y=w263:i32)
              n124 = Subtract(x=w269, y="Main ROI Decay\nper Fail (Vertical)") -> (x-y=w265:i32)
            }
            frame True {
              # "Scale / Score"
              # "Main ROI"
              # "Horizontal Scale \n(smaller number = smaller ROI)"
              n125 = Subtract(x=w304, y=w301) -> (x-y=w300:dbl)
              n126 = Subtract(x=w303, y=w302) -> (x-y=w299:dbl)
              n127 = Add(x=w302, y=w303) -> (x+y=w298:dbl)
              n128 = Array To Cluster(array=w287) -> (cluster=w297:T13)
              n129 = Unbundle By Name(w297) -> ("Matches (Geometric Matching 1)[0].Position.x"=w291:sgl, "Matches (Geometric Matching 1)[0].Position.y"=w293:sgl, "Matches (Geometric Matching 1)[0].Scale"=w292:sgl)
              n130 = Divide(x=w292, y=w289) -> (x/y=w294:sgl)
              n131 = Multiply(x=w292, y=w288) -> (x*y=w296:sgl)
              n132 = Divide(x=w296, y=sgl 2.0) -> (x/y=w290:sgl)
              n133 = Add(x=w293, y=w294) -> (x+y=w283:sgl)
              n134 = Subtract(x=w293, y=w294) -> (x-y=w285:sgl)
              n135 = Subtract(x=w291, y=w290) -> (x-y=w286:sgl)
              n136 = Add(x=w290, y=w291) -> (x+y=w284:sgl)
            }
          }
          n137 = call "Bound_RO_L_R0I.vi"("Bottom Right - Y"=w241, "Right - X"=w242, "Top Left - Y"=w243, "Top  Left - x"=w244) -> ("ROI Descriptor"=w245:T2)  [unwired: 7 in]
        }
      }
      "Next Main ROI Descriptor" <- w38
      n138 = And(x="Startup Flag", y=w82) -> (x .and. y?=w85:bool)
      n139 = case shown="True" w85 {
        tunnel: "Startup Flag" -> [w218 _]
        tunnel: [w218 FALSE] -> w84
        frame False {
        }
        frame True {
        }
      }
      "Startup Flag - out" <- w84
      n140 = Less?(x=w88, y="Absolute\nMinimum Score") -> (x < y?=w92:bool)
      n141 = Less?(x=w51, y="Absolute\nMinimum Scale") -> (x < y?=w54:bool)
      n142 = Greater?(x=w52, y="Absolute\nMaximum Scale") -> (0:w49:bool)
      n143 = Greater?(x=w51, y=w52) -> (0:w55:bool)
      n144 = Less?(x=w52, y=w51) -> (x < y?=w50:bool)
      n145 = Select(t="Absolute\nMinimum Score", s=w92, f=w88) -> (s? t:f=w94:dbl)
      "New Min Score" <- w94
      n146 = Or(x=w54, y=w55) -> (x .or. y?=w56:bool)
      n147 = Or(x=w49, y=w50) -> (x .or. y?=w53:bool)
      n148 = Select(t="Absolute\nMinimum Scale", s=w56, f=w51) -> (s? t:f=w72:dbl)
      "New Low Scale" <- w72
      n149 = Select(t="Absolute\nMaximum Scale", s=w53, f=w52) -> (s? t:f=w73:dbl)
      "New high Scale" <- w73
      n150 = Bundle("index"=w90, "Min Scale"=w72, "Max Scale"=w73) -> (w89:T17)  [unwired: 1 in]
      n151 = Replace Array Subset(array=w87, new element=w89, index=w90) -> (w91:T8[])
      n152 = call "IMAQ Overlay ROI"("ROI Descriptor"=w38, "Image"=w71) -> ("Image Out"=→"Right Image 2":T5)  [unwired: 8 in, 1 out]
      n153 = Bundle By Name(cluster="Current Settings", "Range Settings"=w91, "Minimum Match Score"=w94) -> (→"New Settings":T9)
    }
  }
